vi "Choreo_Choreo_DifferentialRamseteController.vi"(8 "Auto":bool=TRUE, 10 "ChoreoDifferentialSample":T6={"timestamp"=-999.0, "x"=0.0, "y"=0.0, "heading"=0.0, "velocityL"=0.0, "velocityR"=0.0, "angularVelocity"=0.0, "accelL"=0.0, "accelR"=0.0, "accelAngular"=0.0, "forceL"=0.0, "forceR"=0.0}, 11 "Current Position":T3={"TRANSLATION"={"X"=0.0, "Y"=0.0}, "ROTATION"={"VALUE"=0.0, "COS"=1.0, "SIN"=0.0}} {"ROTATION"."SIN" format="%13.4f"; "ROTATION"."COS" format="%13.4f"; "ROTATION"."VALUE" format="%13.4f"; "TRANSLATION"."Y" format="%14.3f"; "TRANSLATION"."X" format="%14.3f"}) -> (2 "On Target":bool, 3 "Chassis Speed Dmd":T2 {"vOmega" format="%10.3f"; "vY" format="%10.3f"; "vX" format="%10.3f"}, 4 "Ctrl Info":T1)   [LabVIEW 2019, in "ChoreoLib.lvlib"]
doc: "Creates and executes a differential drive control function to execute a Choreo Trajectory sample. The controller consists of Ramsete controller.\n\nInputs:\n - Current Pose - pose2d - Current robot position pose calcualted by either Odometry or Pose Estimation.\n - ChoreoTrajectoryState - cluster - Trajectory state to execute\n - Auto - boolean - When TRUE closed loop control is used to control trajectory execution. This is mostly for debugging and robot tuning. (Optional. Default: TRUE )\n\nOutputs:\n - Choreo Speed Demand - chassis speed - Desired chassis speed (M/S, Rad/Sec)\n - On Target - boolean - TRUE when robot position is within tolerance of trajectory position\n - Ctrl Info - cluster - Information on control. Mostly for diagnostics."
uses:
  ChoreoLib.lvlib
  <vilib>/Rock Robotics/WPI/ThirdParty/JAS_Junk/TrajLib/Trajectory_Library.lvlib
  <vilib>/Rock Robotics/WPI/ThirdParty/JAS_Junk/TrajLib/TypeDef/TRANSLATION2D.ctl
  <vilib>/Rock Robotics/WPI/ThirdParty/JAS_Junk/TrajLib/TypeDef/ROTATION2D.ctl
  <vilib>/Rock Robotics/WPI/ThirdParty/JAS_Junk/TrajLib/TypeDef/POSE2D.ctl
  <vilib>/Rock Robotics/WPI/ThirdParty/JAS_Junk/TrajLib/TypeDef/CHASSIS_SPEEDS.ctl
  TypeDef/ChoreoDifferentialSample.ctl
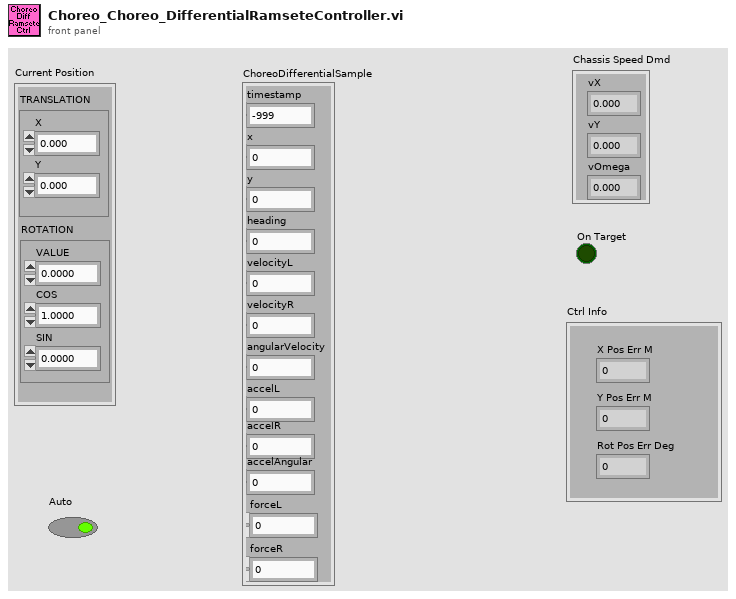
[diagram p1: front panel]
types:
  T1 = cluster{"X Pos Err M":dbl, "Y Pos Err M":dbl, "Rot Pos Err Deg":dbl}
  T2 = typedef "Trajectory_Library.lvlib/CHASSIS_SPEEDS.ctl" = cluster{"vX":dbl, "vY":dbl, "vOmega":dbl}
  T3 = typedef "Trajectory_Library.lvlib/POSE2D.ctl" = cluster{"TRANSLATION":T4, "ROTATION":T5}
  T4 = typedef "Trajectory_Library.lvlib/TRANSLATION2D.ctl" = cluster{"X":dbl, "Y":dbl}
  T5 = typedef "Trajectory_Library.lvlib/ROTATION2D.ctl" = cluster{"VALUE":dbl, "COS":dbl, "SIN":dbl}
  T6 = typedef "ChoreoLib.lvlib/ChoreoDifferentialSample.ctl" = cluster{"timestamp":dbl, "x":dbl, "y":dbl, "heading":dbl, "velocityL":dbl, "velocityR":dbl, "angularVelocity":dbl, "accelL":dbl, "accelR":dbl, "accelAngular":dbl, "forceL":dbl, "forceR":dbl}
  T7 = typedef "Trajectory_Library.lvlib/RAMSETE.ctl" = cluster{"B":dbl, "Zeta":dbl, "poseTolerance":T3, "poseError":T3, "Enabled":bool}
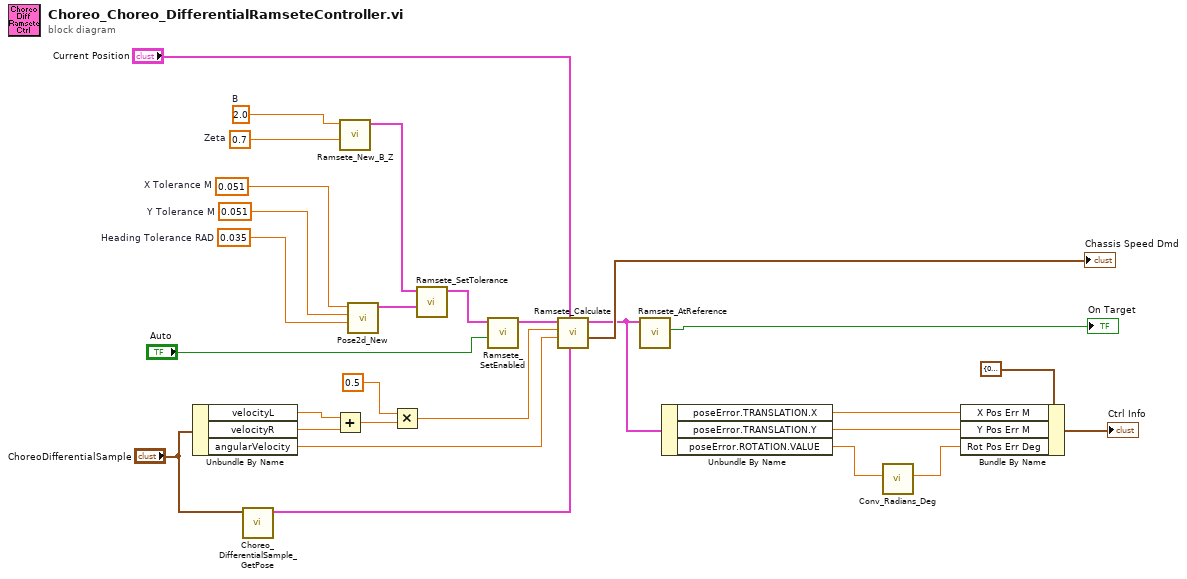
[diagram p0: block diagram]
diagram:
  w20 = 0.051  # X Tolerance M
  w19 = 0.051  # Y Tolerance M
  w22 = 0.7  # Zeta
  w18 = 0.035  # Heading Tolerance RAD
  w23 = 2.0  # B
  n1 = Unbundle By Name("ChoreoDifferentialSample") -> ("velocityL"=w7:dbl, "velocityR"=w6:dbl, "angularVelocity"=w1:dbl)
  n2 = call "Choreo_DifferentialSample_GetPose.vi"("ChoreoDifferentialSample"="ChoreoDifferentialSample") -> ("Pose"=w8:T3)  [unwired: 10 in]
  n3 = Add(x=w7, y=w6) -> (x+y=w5:dbl)
  n4 = call <vilib>:"Ramsete_New_B_Z.vi"("Zeta"=w22, "B"=w23) -> ("outRAMSETE"=w25:T7)  [unwired: 9 in]
  n5 = call <vilib>:"Pose2d_New.vi"("Heading"=w18, "Y"=w19, "X"=w20) -> ("out POSe"=w17:T3)  [unwired: 8 in]
  n6 = Multiply(x=0.5, y=w5) -> (x*y=w2:dbl)
  n7 = call <vilib>:"Ramsete_SetTolerance.vi"("tolerancePose"=w17, "inRAMSETE"=w25) -> ("outRAMSETE"=w24:T7)  [unwired: 9 in]
  n8 = call <vilib>:"Ramsete_SetEnabled.vi"("Enabled"="Auto", "inRAMSETE"=w24) -> ("outRAMSETE"=w15:T7)  [unwired: 9 in]
  n9 = call <vilib>:"Ramsete_Calculate.vi"("DesiredPOSE"=w8, "CurrentPOSE"="Current Position", "DesiredAngularVelocity"=w1, "DesiredLinearVelocity"=w2, "inRAMSETE"=w15) -> ("CHASSIS Speeds"=→"Chassis Speed Dmd":T2, "outRAMSETE"=w12:T7)  [unwired: 5 in]
  n10 = call <vilib>:"Ramsete_AtReference.vi"("RAMSETE"=w12) -> ("AtReference"=→"On Target":bool)  [unwired: 10 in]
  n11 = Unbundle By Name(w12) -> ("poseError.TRANSLATION.X"=w11:dbl, "poseError.TRANSLATION.Y"=w10:dbl, "poseError.ROTATION.VALUE"=w9:dbl)
  n12 = call <vilib>:"Conv_Radians_Deg.vi"("Radians"=w9) -> ("Degrees"=w28:dbl)  [unwired: 10 in]
  n13 = Bundle By Name(cluster=T1 {"X Pos Err M"=0.0, "Y Pos Err M"=0.0, "Rot Pos Err Deg"=0.0} ("Ctrl Info"), "X Pos Err M"=w11, "Y Pos Err M"=w10, "Rot Pos Err Deg"=w28) -> (→"Ctrl Info":T1)
